vi "Write Single Coil.vi"(7 "unit ID":u8, 8 "error in":errorcluster, 9 "coil to write":bool, 10 "address":u16, 11 "Modbus master in":refnum<class "Modbus Master.lvclass">) -> (0 "error out":errorcluster, 3 "Modbus master out":refnum<class "Modbus Master.lvclass">)   [LabVIEW 2013, in "Modbus Library - Advance.lvlib" / "Modbus Master.lvclass"]
doc: "Writes <B>coil to write</B> to <B>address</B> of the device."
uses:
  Modbus Master.lvclass
  Modbus Master.lvclass/Modbus Master.ctl
  Modbus API.lvclass/Modbus API.ctl
  Transmission Data Unit/Transmission Data Unit.lvclass/Transmission Data Unit.ctl
  Transmission Data Unit/Transmission Data Unit.lvclass
  Master Function Definition/Master Function Definition.lvclass
  Modbus API.lvclass
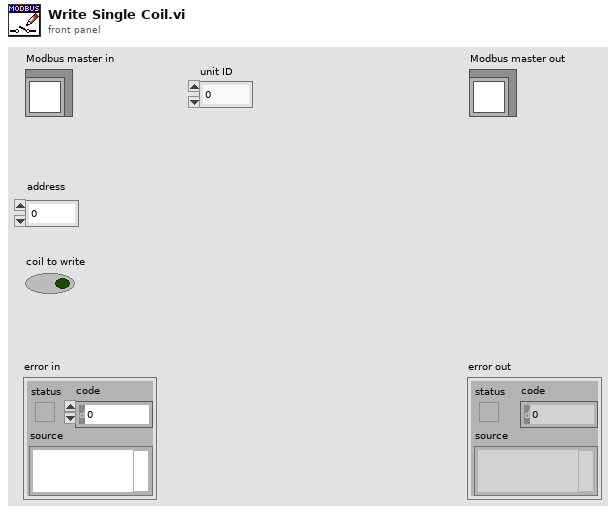
[diagram p1: front panel]
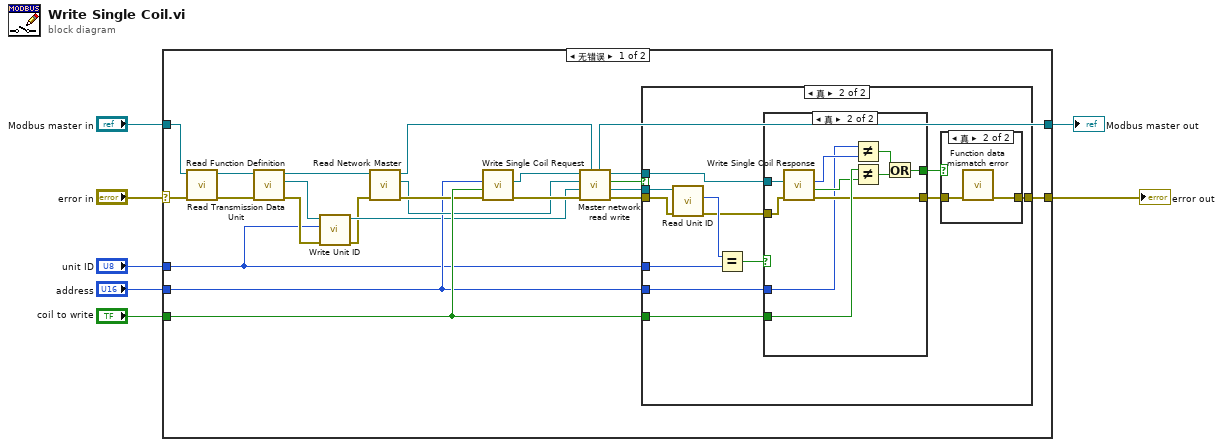
[diagram p0: block diagram]
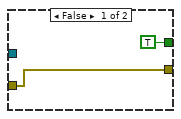
[diagram p3: hidden frame]
diagram:
  n1 = case shown="无错误" "error in" {
    selector: "error in" -> [w20 w60]
    tunnel: "Modbus master in" -> [w19 w59]
    tunnel: [w29 w60] -> w4
    tunnel: [w24 w59] -> w3
    tunnel: "address" -> [w15 _]
    tunnel: "coil to write" -> [w28 _]
    tunnel: "unit ID" -> [w9 _]
    frame No Error {
      n2 = call "Read Function Definition.vi"("error in"=w20, "Modbus master in"=w19) -> ("error out"=w22:errorcluster, "Modbus master out"=w21:refnum<class "Modbus Master.lvclass">)  [unwired: 7 in, 1 out]
      n3 = call "Read Transmission Data Unit.vi"("error in"=w22, "Modbus instance in"=w21) -> ("error out"=w11:errorcluster, "transmission data unit"=w13:refnum<class "Transmission Data Unit.lvclass">, "Modbus instance out"=w23:refnum<class "Modbus Master.lvclass">)  [unwired: 7 in]
      n4 = call "Write Unit ID.vi"("error in"=w11, "unit ID"=w9, "transmission data unit in"=w13) -> ("error out"=w10:errorcluster, "transmission data unit out"=w12:refnum<class "Transmission Data Unit.lvclass">)  [unwired: 7 in]
      n5 = call "Read Network Master.vi"("error in"=w10, "Modbus master in"=w23) -> ("error out"=w18:errorcluster, "network master"=w16:refnum<class "Network Master.lvclass">, "Modbus master out"=w17:refnum<class "Modbus Master.lvclass">)  [unwired: 7 in]
      n6 = call "Write Single Coil Request.vi"("error in"=w18, "Coil Value"=w28, "Starting Address"=w15) -> ("error out"=w30:errorcluster, "modbus data unit out"=w26:refnum<class "Modbus Data Unit.lvclass">)  [unwired: 7 in]
      n7 = call "Master network read write.vi"("Modbus master in"=w17, "error in"=w30, "transmission data unit in"=w12, "network master in"=w16, "Modbus data unit in"=w26) -> ("error out"=w27:errorcluster, "transmission data unit out"=w8:refnum<class "Transmission Data Unit.lvclass">, "PDU Valid?"=w14:bool, "Modbus data unit out"=w25:refnum<class "Modbus Data Unit.lvclass">, "Modbus master out"=w24:refnum<class "Modbus Master.lvclass">)  [unwired: 2 in]
      n8 = case shown="真" w14 {
        tunnel: [w31 w42] -> w29
        tunnel: w28 -> [_ w41]
        tunnel: w27 -> [w31 w36]
        tunnel: w25 -> [_ w40]
        tunnel: w15 -> [_ w38]
        tunnel: w9 -> [_ w34]
        tunnel: w8 -> [_ w37]
        frame False {
        }
        frame True {
          n9 = call "Read Unit ID.vi"("error in"=w36, "transmission data unit in"=w37) -> ("error out"=w32:errorcluster, "unit ID"=w35:u8)  [unwired: 7 in, 1 out]
          n10 = Equal?(x=w35, y=w34) -> (x = y?=w33:bool)
          n11 = case shown="真" w33 {
            tunnel: [TRUE w55] -> w43
            tunnel: w41 -> [_ w51]
            tunnel: w40 -> [_ w49]
            tunnel: [w45 w48] -> w39
            tunnel: w38 -> [_ w47]
            tunnel: w32 -> [w45 w46]
            frame False {
            }
            frame True {
              n12 = call "Write Single Coil Response.vi"("error in"=w46, "modbus data unit in"=w49) -> ("error out"=w48:errorcluster, "Coil Value"=w50:bool, "Address"=w52:u16)  [unwired: 7 in]
              n13 = Not Equal?(x=w47, y=w52) -> (x != y?=w54:bool)
              n14 = Not Equal?(x=w51, y=w50) -> (x != y?=w53:bool)
              n15 = Or(x=w54, y=w53) -> (x .or. y?=w55:bool)
            }
          }
          n16 = case shown="真" w43 {
            tunnel: [w56 w58] -> w42
            tunnel: w39 -> [w56 w57]
            frame False {
            }
            frame True {
              n17 = call "Function data mismatch error.vi"("error in (no error)"=w57) -> ("error out"=w58:errorcluster)  [unwired: 10 in]
            }
          }
        }
      }
    }
    frame Error {
    }
  }
  "error out" <- w4
  "Modbus master out" <- w3
